vi "TestDataSendCloud.vi"() -> ()   [LabVIEW 2017]
panel:
  out "MainConfigurationArray":cluster{"Parameter":string, "Value":string}[](array[cluster])
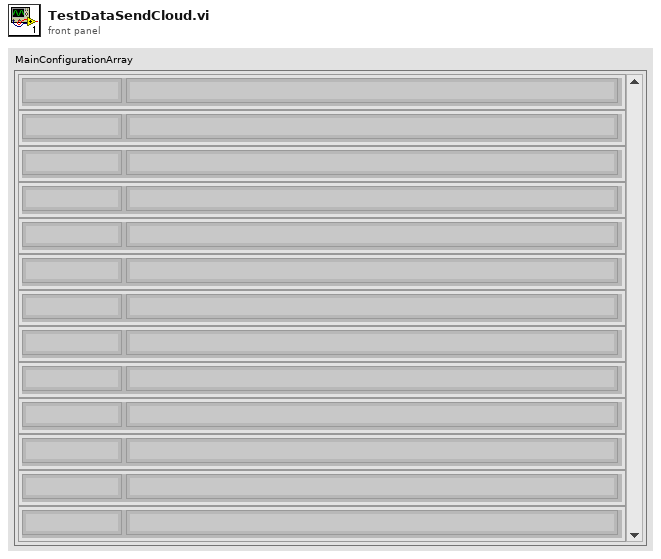
[diagram p1: front panel]
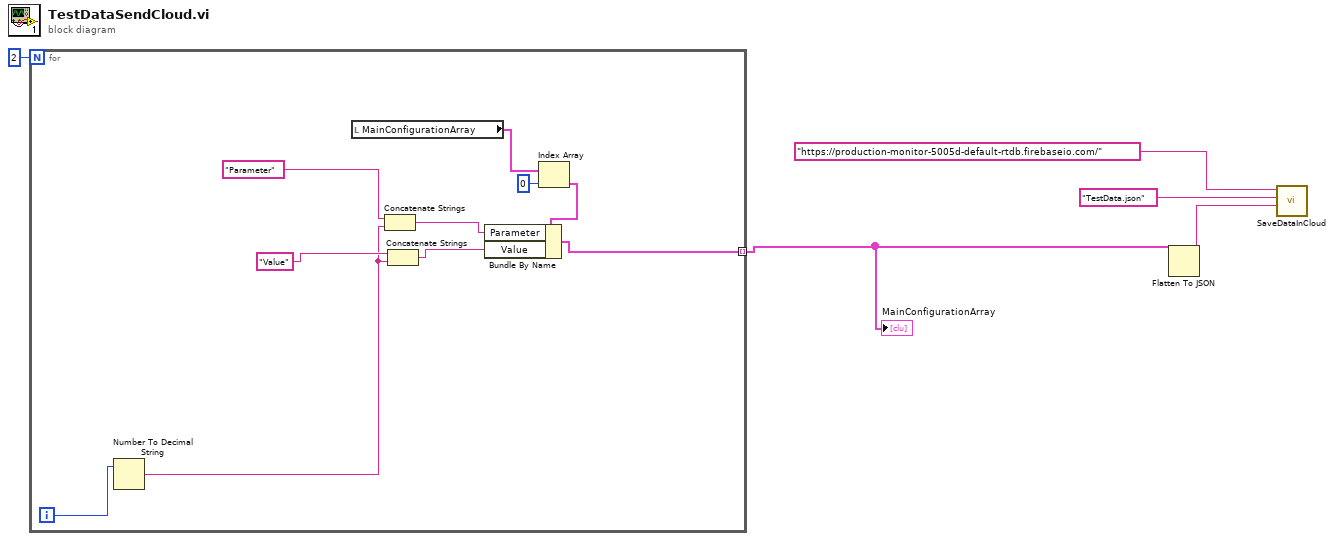
[diagram p0: block diagram]
diagram:
  n1 = for {
    N: 2 -> [_]
    tunnel: [w6] -> w1 mode=indexing
    i -> [w15]
    n2 = Number To Decimal String(number=w15) -> (decimal integer string=w12:string)  [unwired: 1 in]
    n3 = local read "MainConfigurationArray"() -> (w11:cluster{"Parameter":string, "Value":string}[])
    n4 = Concatenate Strings("Parameter", w12) -> (w7:string)
    n5 = Concatenate Strings("Value", w12) -> (w8:string)
    n6 = Index Array(array=w11, index=0) -> (element=w9:cluster{"Parameter":string, "Value":string})
    n7 = Bundle By Name(cluster=w9, "Parameter"=w7, "Value"=w8) -> (w6:cluster{"Parameter":string, "Value":string})
  }
  "MainConfigurationArray" <- w1
  n8 = Flatten To JSON(anything=w1) -> (JSON string=w2:string)  [unwired: 2 in, 1 out]
  n9 = call "SaveDataInCloud.vi"("DataToBeStored"=w2, "FileName"="TestData.json", "CloudAddress"="https://production-monitor-5005d-default-rtdb.firebaseio.com/") -> ()  [unwired: 9 in]
